vi "S2C_UNITHERM_Proc_Status.vi"(8 "Error In":errorcluster) -> (0 "Error Out":errorcluster, 3 "Response":string)   [LabVIEW 2024]
uses:
  S2C_UNITHERM_Proc_Globals.vi
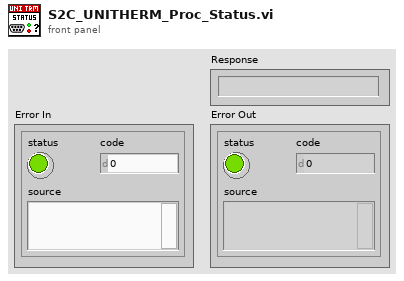
[diagram p1: front panel]
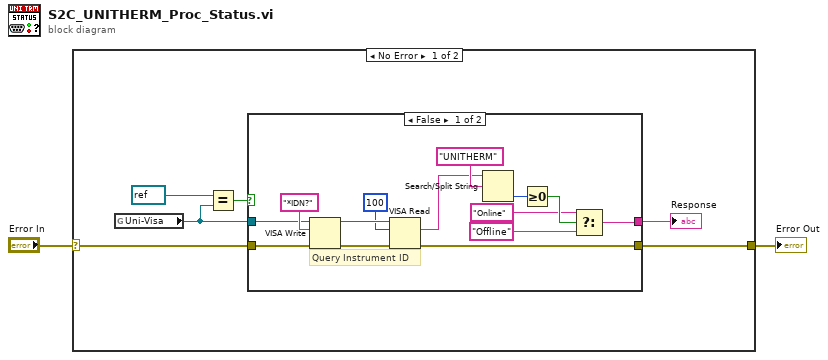
[diagram p0: block diagram]
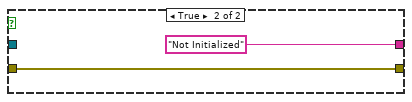
[diagram p2: hidden frame]
diagram:
  n1 = case shown="No Error" "Error In" {
    selector: "Error In" -> [w8 w25]
    tunnel: [w7 w25] -> w1
    frame No Error {
      n2 = global read "S2C_UNITHERM_Proc_Globals.vi" "Uni-Visa"() -> (w3:refnum<visa-resource-name>)
      n3 = Equal?(x=refnum<visa-resource-name> refnum ("SerialRef"), y=w3) -> (x = y?=w4:bool)
      n4 = case shown="False" w4 {
        tunnel: w8 -> [w18 w24]
        tunnel: w3 -> [w17 _]
        tunnel: [w10 w24] -> w7
        tunnel: [w9 "Not Initialized" ("f")] -> w6
        frame False {
          # "Query Instrument ID"
          n5 = VISA Write(VISA resource name=w17, write buffer="*IDN?", error in (no error)=w18) -> (VISA resource name out=w22:refnum<visa-resource-name>, error out=w20:errorcluster)  [unwired: 1 out]
          n6 = VISA Read(VISA resource name=w22, byte count=u32 100, error in (no error)=w20) -> (read buffer=w14:string, error out=w10:errorcluster)  [unwired: 2 out]
          n7 = Search/Split String(string=w14, search string/char (-)="UNITHERM") -> (offset of match=w15:i32)  [unwired: 1 in, 2 out]
          n8 = Greater Or Equal To 0?(x=w15) -> (x >= 0?=w13:bool)
          n9 = Select(t="Online", s=w13, f="Offline") -> (s? t:f=w9:string)
        }
        frame True {
        }
      }
      "Response" <- w6
    }
    frame Error {
    }
  }
  "Error Out" <- w1
